vi "Write Launch Notifier.vi"(8 "error in (no error)":errorcluster, 10 "Launch Notifier":refnum<notifier>, 11 "Measure Controller in":refnum<class "Process Controller.lvclass">) -> (0 "error out":errorcluster, 3 "Measure Controller out":refnum<class "Process Controller.lvclass">)   [LabVIEW 2016, in "Process Controller.lvclass"]
uses:
  Process Controller.lvclass
  Process Controller.lvclass/Process Controller.ctl
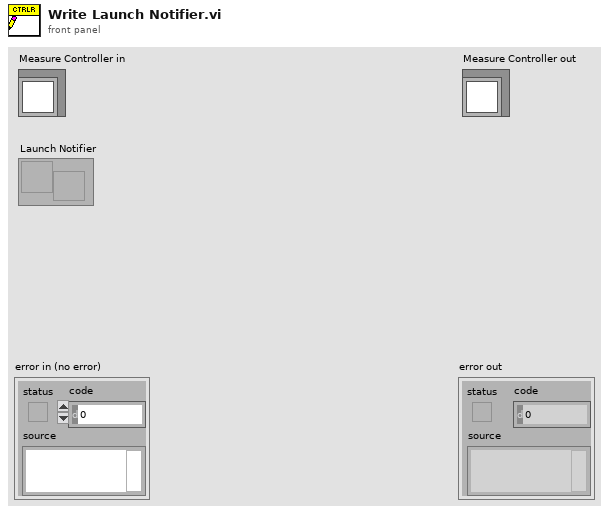
[diagram p1: front panel]
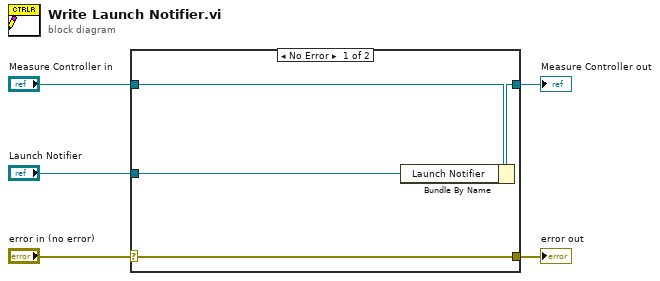
[diagram p0: block diagram]
diagram:
  n1 = case shown="No Error" "error in (no error)" {
    selector: "error in (no error)" -> [w9 w10]
    tunnel: [w9 w10] -> w4
    tunnel: [w7 w11] -> w2
    tunnel: "Measure Controller in" -> [w8 w11]
    tunnel: "Launch Notifier" -> [w6 _]
    frame No Error {
      n2 = Bundle By Name(cluster=w8, "Launch Notifier"=w6) -> (w7:refnum<class "Process Controller.lvclass">)
    }
    frame Error {
    }
  }
  "error out" <- w4
  "Measure Controller out" <- w2
